vi "RandomNumberSubVI.vi"(8 "Maximum":dbl, 11 "Minimum":dbl) -> (3 "Random Number":dbl)   [LabVIEW 2018]
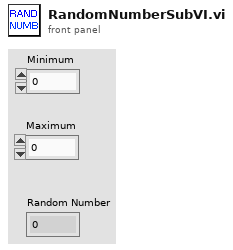
[diagram p1: front panel]
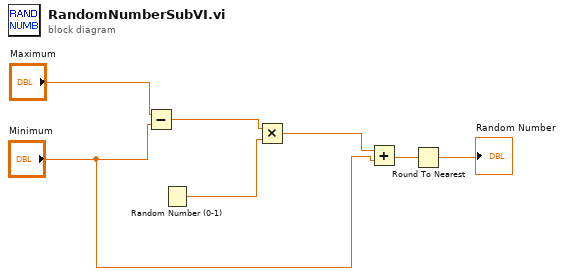
[diagram p0: block diagram]
diagram:
  n1 = Subtract(x="Maximum", y="Minimum") -> (x-y=w6:dbl)
  n2 = Random Number (0-1)() -> (number: 0 to 1=w5:dbl)
  n3 = Multiply(x=w6, y=w5) -> (x*y=w4:dbl)
  n4 = Add(x=w4, y="Minimum") -> (x+y=w2:dbl)
  n5 = Round To Nearest(number=w2) -> (nearest integer value=→"Random Number":dbl)
